vi "bats.parser.hostToFpga.testRunner.vi"(9 "Test.Messages":variant[](array[variant]), 10 "Expected OrderBook.Command[]":T1[](array[typedef])) -> (0 "Failures.Count":i32=1, 1 "Actual [str]":string[](array[string]), 2 "Passed":bool, 3 "OrderBook.Command[]":T1[](array[typedef]), 4 "Debug":u64[](array[numeric]) format="%.0x", 5 "Expected [str]":string[](array[string]))   [LabVIEW 2020]
uses:
  Market.Data.Common/fpga/orderbook.command.ctl
  Market.Data.Common/fpga/orderbook.command.type.ctl
  <vilib>/rvi/interface/RandomDataEmulation/nirviRandomDataOpen.vi
  <vilib>/rvi/interface/common/niFpgaCacheSessionInfoDynamic.vi
  <vilib>/Utility/error.llb/Error Cluster From Error Code.vi
  <vilib>/rvi/errors/niLvFpgaAdjustHostInterfaceError.vi
  <vilib>/FPGAPlugInAG/Dynamic/niLvFpga_Close_Dynamic.vi
  <vilib>/rvi/interface/nirviOpenFPGA/nirviOpenFPGA.xnode
  fpga/bats.parser.test.vi
  <vilib>/rvi/interface/nirviReadWriteControl/nirviReadWriteControl.xnode
  <vilib>/rvi/interface/nirviMethod/nirviMethod.xnode
  <vilib>/rvi/interface/nirviCloseFPGA/nirviCloseFPGA.xnode
  <vilib>/rvi/errors/niLvFpgaMergeErrorWithErrorCode.vi
  <vilib>/FPGAPlugInAG/Dynamic/niLvFpga_ReadFifo_Dynamic.vi
  <vilib>/rvi/interface/Simulation/niFpgaSimulationCallBeginRW.vi
  Market.Data.Common/host/fpganow.common.host.lvlib
  NiFpgaLv.dll
  <vilib>/FPGAPlugInAG/Dynamic/niLvFpga_WriteFifo_Dynamic.vi
  Market.Data.Common/fpga/fpganow.common.fpga.lvlib
panel:
  out "size(s)":i32
  out "Words.Out":u16[](array[numeric]) format="%.0x"
  out "Data.size":i32=16
  in  "Execute?":bool=TRUE
  out "Data":u64[](array[numeric]) format="%.0x"
  out "error out":errorcluster
  in  "error in":errorcluster
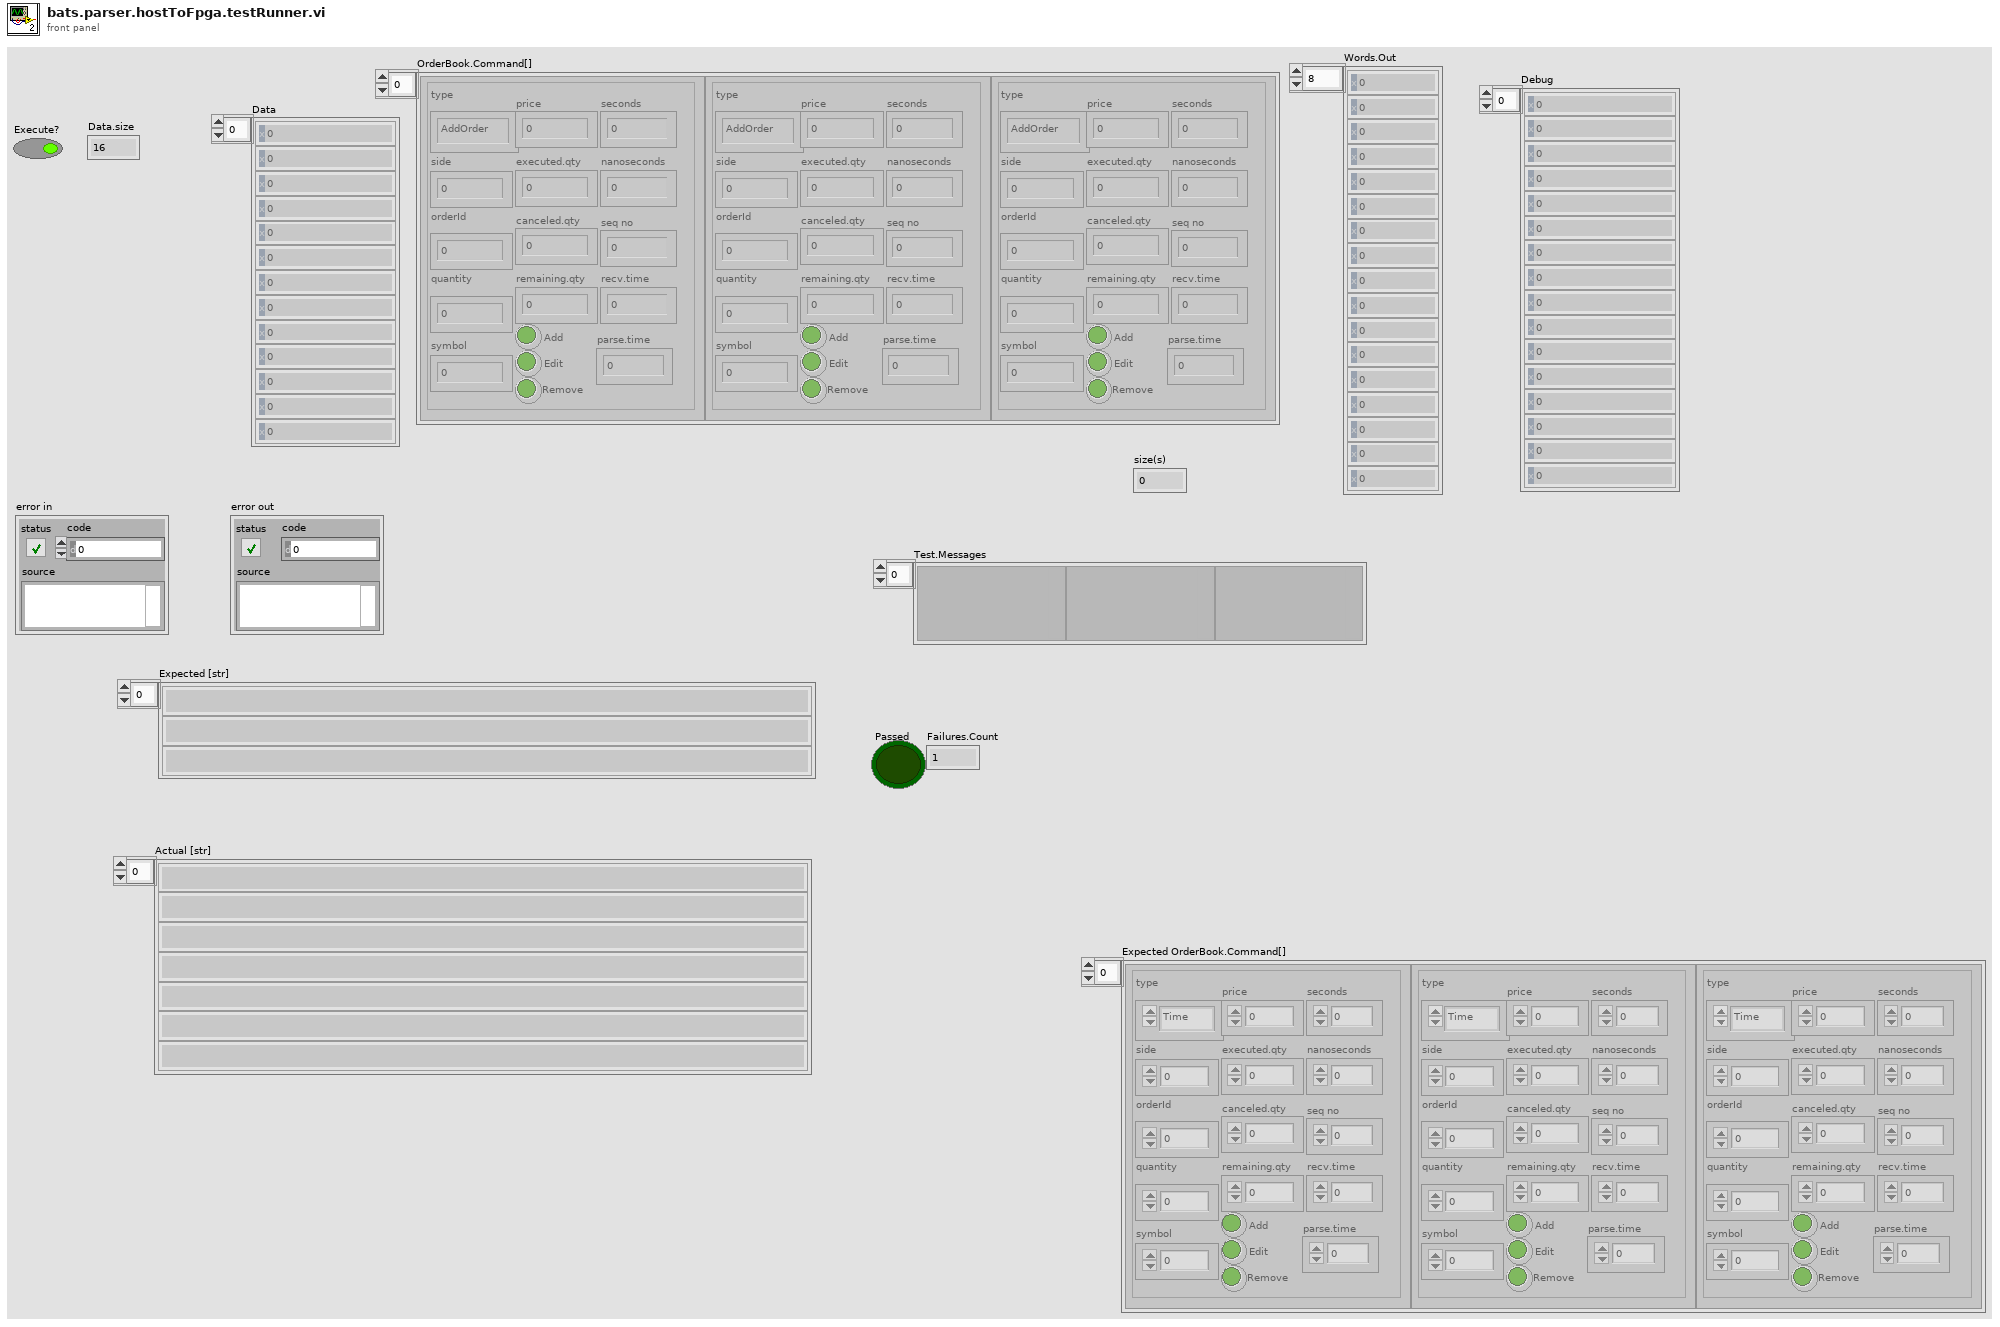
[diagram p1: front panel]
types:
  T1 = typedef "fpganow.common.fpga.lvlib/orderbook.command.ctl" = cluster{"type":T2, "side":u8, "orderId ":u64, "quantity":u32, "symbol":u64, "price":u64, "executed.qty":u32, "canceled.qty":u32, "remaining.qty":u32, "seconds":u64, "nanoseconds":u64, "Add":bool, "Edit":bool, "Remove":bool, "seq no":u32, "recv.time":u64, "parse.time":u64}
  T2 = typedef "fpganow.common.fpga.lvlib/orderbook.command.type.ctl" = enum8{"Time", "AddOrder", "OrderExecuted", "OrderExecutedAtPrice", "ReduceSize", "ModifyOrder", "DeleteOrder", "Get.Everything", "Get.All.Orders", "Get.Top"}
  T3 = cluster{"type":bool, "side":bool, "orderId ":bool, "quantity":bool, "symbol":bool, "price":bool, "executed.qty":bool, "canceled.qty":bool, "remaining.qty":bool, "seconds":bool, "nanoseconds":bool, "Add":bool, "Edit":bool, "Remove":bool, "seq no":bool, "recv.time":bool, "parse.time":bool}
  T4 = cluster{"Index":i32, "x = y?":cluster{"type":bool, "side":bool, "orderId ":bool, "quantity":bool, "symbol":bool, "price":bool, "executed.qty":bool, "canceled.qty":bool, "remaining.qty":bool, "seconds":bool, "nanoseconds":bool, "Add":bool, "Edit":bool, "Remove":bool, "seq no":bool, "recv.time":bool, "parse.time":bool}}
  T5 = cluster{"Index":i32, "x = y?":cluster{"type":bool, "side":bool, "orderId ":bool, "quantity":bool, "symbol":bool, "price":bool, "executed.qty":bool, "canceled.qty":bool, "remaining.qty":bool, "seconds":bool, "nanoseconds":bool, "Add":bool, "Edit":bool, "Remove":bool, "seq no":bool, "recv.time":bool, "parse.time":bool}}[]
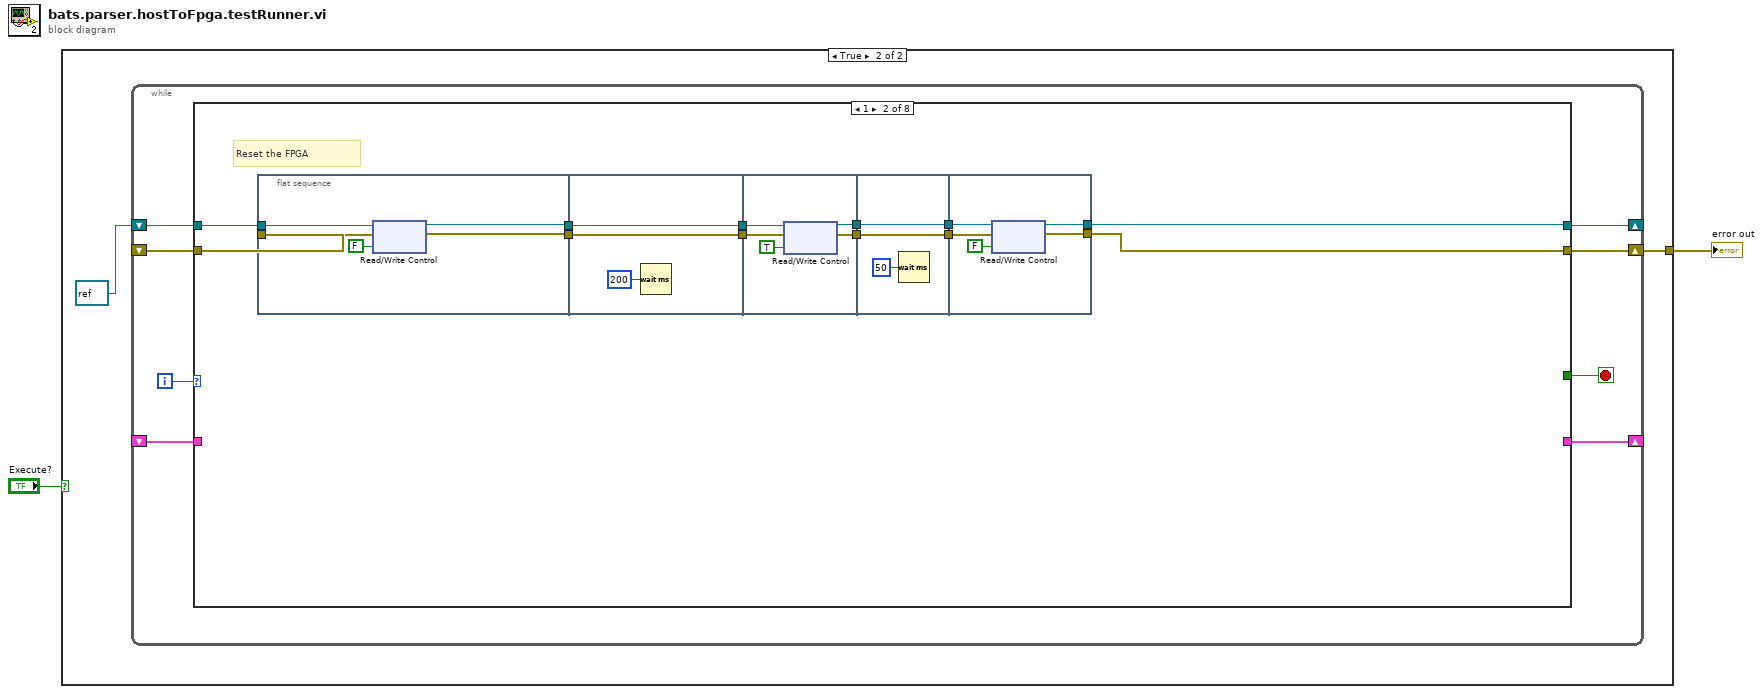
[diagram p0: block diagram]
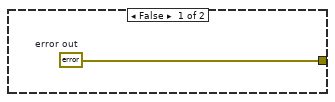
[diagram p2: hidden frame]
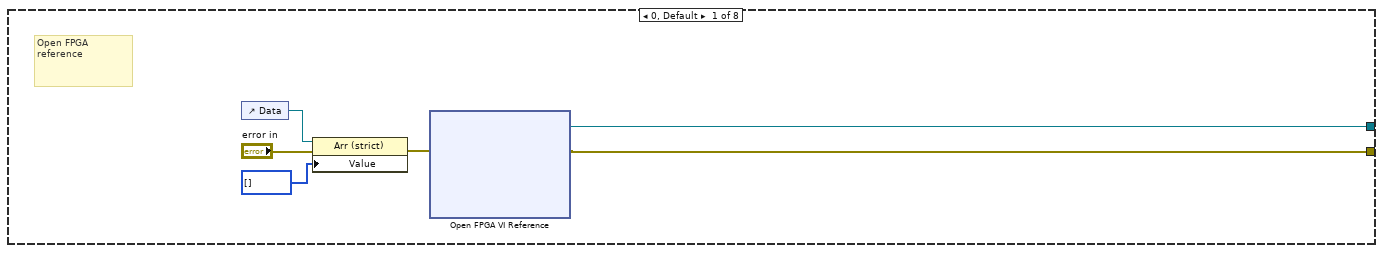
[diagram p3: hidden frame]
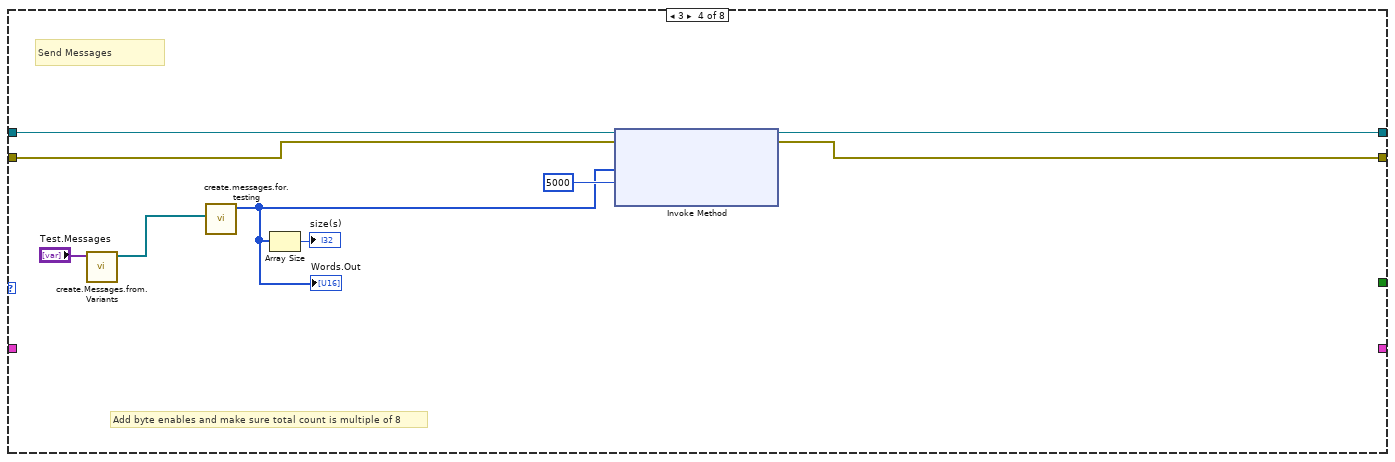
[diagram p5: hidden frame]
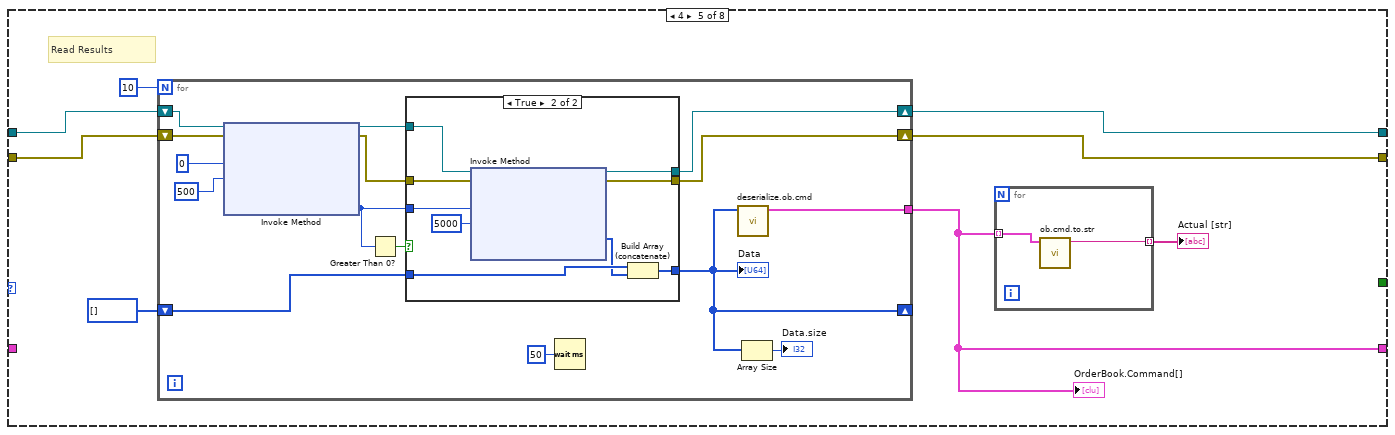
[diagram p6: hidden frame]
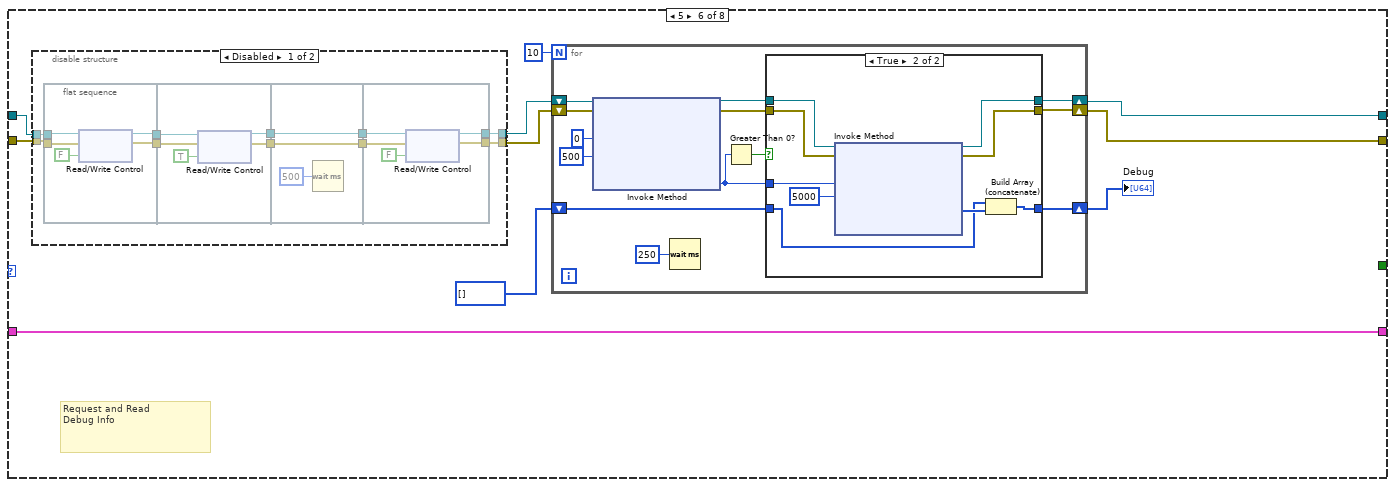
[diagram p8: hidden frame]
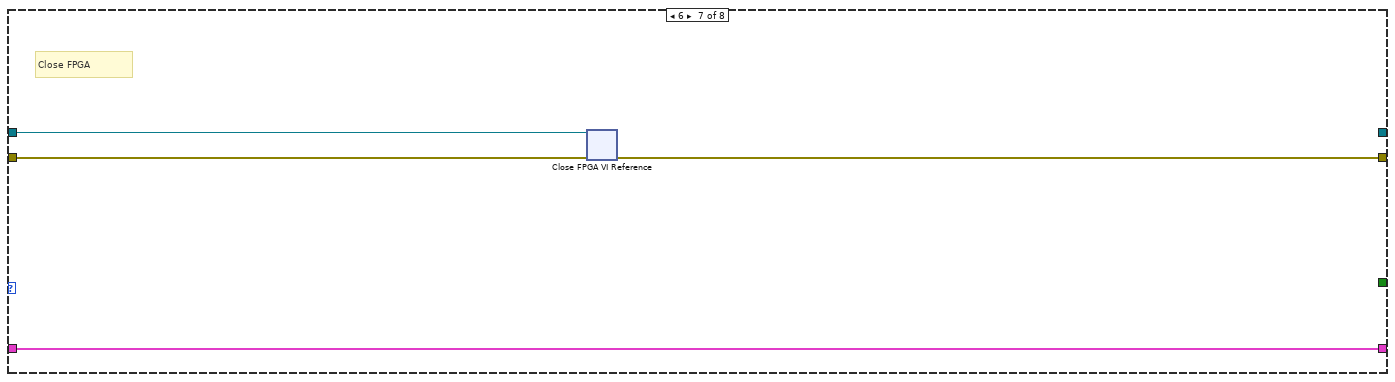
[diagram p11: hidden frame]
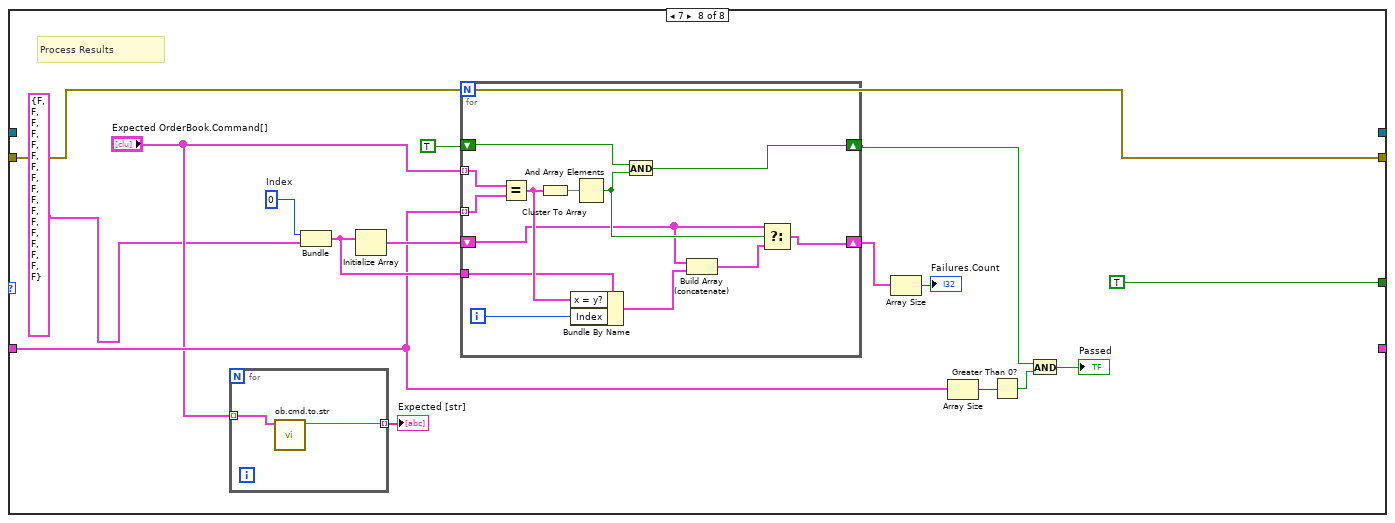
[diagram p12: hidden frame]
diagram:
  n1 = case shown="True" "Execute?" {
    tunnel: [w3 w5] -> w2
    frame False {
      w3 = errorcluster {"status"=FALSE, "code"=0, "source"=""}  # error out
    }
    frame True {
      n2 = while {
        shift-right: [w11] -> _
        shift-left: refnum<k20> refnum ("FPGA VI Reference Out") -> [w9]
        shift-right: [w10] -> w5
        shift-left: _ -> [w8]
        shift-right: [w7] -> _
        shift-left: _ -> [w6]
        i -> [w13]
        stop <- w12 stop-if-true
        n3 = case shown="1" w13 {
          tunnel: [_ _ _ _ _ _ _ TRUE] -> w12
          tunnel: [w14 w24 w54 w60 w66 w105 _ _] -> w11
          tunnel: [w15 w25 w53 w59 w67 w106 w169 w173] -> w10
          tunnel: w9 -> [_ w27 w54 w62 w69 w109 w168 _]
          tunnel: w8 -> [_ w26 w53 w61 w68 w110 w167 w173]
          tunnel: [_ _ _ _ w65 w101 w166 _] -> w7
          tunnel: w6 -> [_ _ _ _ _ w101 w166 w174]
          frame 0, Default {
            # "Open FPGA\nreference"
            n4 = control-ref of="Data"() -> (w17:refnum<vi>)
            n5 = property class="Arr (strict)"(reference=w17, error in="error in", "Value"=u8[] []) -> (error out=w19:errorcluster)  [unwired: 1 out]
            n6 = xnode ("Open FPGA VI Reference")("error in"=w19) -> ("FPGA VI Reference Out"=w14:refnum<k20>, "error out"=w15:errorcluster)  [unwired: 1 in]
          }
          frame 1 {
            # "Reset the FPGA"
            n7 = flat-sequence {
              tunnel: [w35] -> w23
              tunnel: [w36] -> w21
              tunnel: w27 -> [w33]
              tunnel: w26 -> [w34]
              tunnel: w23 -> [w39]
              tunnel: [w39] -> w22
              tunnel: w21 -> [w38]
              tunnel: [w38] -> w20
              tunnel: [w43] -> w31
              tunnel: [w42] -> w30
              tunnel: w22 -> [w41]
              tunnel: w20 -> [w40]
              tunnel: [w47] -> w29
              tunnel: w31 -> [w47]
              tunnel: w30 -> [w46]
              tunnel: [w46] -> w28
              tunnel: w29 -> [w51]
              tunnel: w28 -> [w50]
              tunnel: [w49] -> w25
              tunnel: [w48] -> w24
              frame #0 {
                n8 = xnode "Read/Write Control"("FPGA VI Reference In"=w33, "error in"=w34, "reset"=FALSE) -> ("FPGA VI Reference Out"=w36:refnum<k20>, "error out"=w35:errorcluster)
              }
              frame #1 {
                n9 = Wait (ms)(milliseconds to wait=u32 200) -> ()  [unwired: 1 out]
              }
              frame #2 {
                n10 = xnode "Read/Write Control"("FPGA VI Reference In"=w40, "error in"=w41, "reset"=TRUE) -> ("FPGA VI Reference Out"=w42:refnum<k20>, "error out"=w43:errorcluster)
              }
              frame #3 {
                n11 = Wait (ms)(milliseconds to wait=u32 50) -> ()  [unwired: 1 out]
              }
              frame #4 {
                n12 = xnode "Read/Write Control"("FPGA VI Reference In"=w50, "error in"=w51, "reset"=FALSE) -> ("FPGA VI Reference Out"=w48:refnum<k20>, "error out"=w49:errorcluster)
              }
            }
          }
          frame 2 {
            # "Memory Configuration"
          }
          frame 3 {
            # "Add byte enables and make sure total count is multiple of 8"
            # "Send Messages"
            n13 = call "create.Messages.from.Variants.vi"("Messages.Variant"="Test.Messages") -> ("Messages"=w56:refnum<class "MessageBase.lvclass">[])  [unwired: 10 in]
            n14 = call "create.messages.for.testing.vi"("Message.to.Create"=w56) -> ("Words.Out"=w58:u16[])  [unwired: 10 in]
            "Words.Out" <- w58
            n15 = Array Size(array=w58) -> (size(s)=→"size(s)":i32)
            n16 = xnode "Invoke Method"("FPGA VI Reference In"=w62, "error in"=w61, "Data"=w58, "Timeout (ms)"=5000) -> ("FPGA VI Reference Out"=w60:refnum<k20>, "error out"=w59:errorcluster)  [unwired: 1 out]
          }
          frame 4 {
            # "Read Results"
            n17 = for {
              N: 10 -> [_]
              shift-right: [w76] -> _
              shift-left: u64[] [] -> [w81]
              shift-right: [w80] -> w66
              shift-left: w69 -> [w88]
              shift-right: [w79] -> w67
              shift-left: w68 -> [w87]
              tunnel: [w74] -> w65
              n18 = xnode "Invoke Method"("FPGA VI Reference In"=w88, "error in"=w87, "Number of Elements"=u32 0, "Timeout (ms)"=500) -> ("FPGA VI Reference Out"=w82:refnum<k20>, "error out"=w78:errorcluster, "Elements Remaining"=w83:u32)  [unwired: 1 out]
              n19 = Greater Than 0?(x=w83) -> (x > 0?=w84:bool)
              n20 = case shown="True" w84 {
                tunnel: w83 -> [_ w100]
                tunnel: w82 -> [w90 w98]
                tunnel: [w91 w95] -> w76
                tunnel: w81 -> [w91 w97]
                tunnel: [w90 w94] -> w80
                tunnel: [w89 w93] -> w79
                tunnel: w78 -> [w89 w92]
                frame False {
                }
                frame True {
                  n21 = xnode "Invoke Method"("FPGA VI Reference In"=w98, "error in"=w92, "Number of Elements"=w100, "Timeout (ms)"=5000) -> ("FPGA VI Reference Out"=w94:refnum<k20>, "error out"=w93:errorcluster, "Data"=w96:u64[])  [unwired: 1 out]
                  n22 = Build Array (concatenate)(w97, w96) -> (w95:u64[])
                }
              }
              "Data" <- w76
              n23 = Wait (ms)(milliseconds to wait=u32 50) -> ()  [unwired: 1 out]
              n24 = call "deserialize.ob.cmd.vi"("DataIn"=w76) -> ("OrderBook.Command[]"=w74:T1[])  [unwired: 10 in]
              n25 = Array Size(array=w76) -> (size(s)=→"Data.size":i32)
            }
            "OrderBook.Command[]" <- w65
            n26 = for {
              tunnel: w65 -> [w73] mode=indexing
              tunnel: [w72] -> w64 mode=indexing
              n27 = call "ob.cmd.to.str.vi"("orderbook.command"=w73) -> ("string"=w72:string)  [unwired: 10 in]
            }
            "Actual [str]" <- w64
          }
          frame 5 {
            # "Request and Read\nDebug Info"
            n28 = disable-structure shown="Disabled" {
              disable-tunnel: w110 -> [w114 w139]
              disable-tunnel: w109 -> [w113 w140]
              disable-tunnel: [w112 w140] -> w108
              disable-tunnel: [w111 w139] -> w107
              frame Disabled {
                n29 = flat-sequence {
                  tunnel: w113 -> [w122]
                  tunnel: w114 -> [w123]
                  tunnel: [w124] -> w120
                  tunnel: [w125] -> w119
                  tunnel: [w129] -> w118
                  tunnel: [w128] -> w117
                  tunnel: w120 -> [w127]
                  tunnel: w119 -> [w126]
                  tunnel: [w133] -> w116
                  tunnel: w118 -> [w133]
                  tunnel: w117 -> [w132]
                  tunnel: [w132] -> w115
                  tunnel: w116 -> [w137]
                  tunnel: w115 -> [w136]
                  tunnel: [w135] -> w111
                  tunnel: [w134] -> w112
                  frame #0 {
                    n30 = xnode "Read/Write Control"("FPGA VI Reference In"=w122, "error in"=w123, "debug"=FALSE ("reset")) -> ("FPGA VI Reference Out"=w125:refnum<k20>, "error out"=w124:errorcluster)
                  }
                  frame #1 {
                    n31 = xnode "Read/Write Control"("FPGA VI Reference In"=w126, "error in"=w127, "debug"=TRUE ("reset")) -> ("FPGA VI Reference Out"=w128:refnum<k20>, "error out"=w129:errorcluster)
                  }
                  frame #2 {
                    n32 = Wait (ms)(milliseconds to wait=u32 500) -> ()  [unwired: 1 out]
                  }
                  frame #3 {
                    n33 = xnode "Read/Write Control"("FPGA VI Reference In"=w136, "error in"=w137, "debug"=FALSE ("reset")) -> ("FPGA VI Reference Out"=w134:refnum<k20>, "error out"=w135:errorcluster)
                  }
                }
              }
              frame Enabled {
              }
            }
            n34 = for {
              N: 10 -> [_]
              shift-right: [w147] -> w105
              shift-left: w108 -> [w153]
              shift-right: [w146] -> w106
              shift-left: w107 -> [w152]
              shift-right: [w148] -> w104
              shift-left: u64[] [] -> [w142]
              n35 = xnode "Invoke Method"("FPGA VI Reference In"=w153, "error in"=w152, "Number of Elements"=u32 0, "Timeout (ms)"=500) -> ("FPGA VI Reference Out"=w145:refnum<k20>, "error out"=w144:errorcluster, "Elements Remaining"=w143:u32)  [unwired: 1 out]
              n36 = Wait (ms)(milliseconds to wait=u32 250) -> ()  [unwired: 1 out]
              n37 = Greater Than 0?(x=w143) -> (x > 0?=w149:bool)
              n38 = case shown="True" w149 {
                tunnel: [w154 w164] -> w148
                tunnel: [w156 w163] -> w147
                tunnel: [w155 w162] -> w146
                tunnel: w145 -> [w156 w161]
                tunnel: w144 -> [w155 w160]
                tunnel: w143 -> [_ w159]
                tunnel: w142 -> [w154 w157]
                frame False {
                }
                frame True {
                  n39 = xnode "Invoke Method"("FPGA VI Reference In"=w161, "error in"=w160, "Number of Elements"=w159, "Timeout (ms)"=5000) -> ("FPGA VI Reference Out"=w163:refnum<k20>, "error out"=w162:errorcluster, "Data"=w165:u64[])  [unwired: 1 out]
                  n40 = Build Array (concatenate)(w157, w165) -> (w164:u64[])
                }
              }
            }
            "Debug" <- w104
          }
          frame 6 {
            # "Close FPGA"
            n41 = xnode "Close FPGA VI Reference"("FPGA VI Reference In"=w168, "error in"=w167) -> ("error out"=w169:errorcluster)
          }
          frame 7 {
            w176 = 0  # Index
            # "Process Results"
            n42 = for {
              tunnel: "Expected OrderBook.Command[]" -> [w187] mode=indexing
              tunnel: [w186] -> w171 mode=indexing
              n43 = call "ob.cmd.to.str.vi"("orderbook.command"=w187) -> ("string"=w186:string)  [unwired: 10 in]
            }
            "Expected [str]" <- w171
            n44 = Bundle("Index"=w176, "x = y?"=T3 {"type"=FALSE, "side"=FALSE, "orderId "=FALSE, "quantity"=FALSE, "symbol"=FALSE, "price"=FALSE, "executed.qty"=FALSE, "canceled.qty"=FALSE, "remaining.qty"=FALSE, "seconds"=FALSE, "nanoseconds"=FALSE, "Add"=FALSE, "Edit"=FALSE, "Remove"=FALSE, "seq no"=FALSE, "recv.time"=FALSE, "parse.time"=FALSE}) -> (w178:T4)  [unwired: 1 in]
            n45 = Initialize Array(w178) -> (w177:T5)  [unwired: 1 in]
            n46 = for {
              tunnel: "Expected OrderBook.Command[]" -> [w200] mode=indexing
              tunnel: w174 -> [w199] mode=indexing
              shift-right: [w197] -> w184
              shift-left: TRUE -> [w198]
              shift-right: [w194] -> w179
              shift-left: w177 -> [w189]
              tunnel: w178 -> [w192]
              i -> [w191]
              n47 = Equal?(x=w200, y=w199) -> (x = y?=w193:T3)
              n48 = Cluster To Array(cluster=w193) -> (array=w196:bool[])
              n49 = Bundle By Name(cluster=w192, "x = y?"=w193, "Index"=w191) -> (w190:T4)
              n50 = And Array Elements(Boolean array=w196) -> (logical AND=w195:bool)
              n51 = And(x=w198, y=w195) -> (x .and. y?=w197:bool)
              n52 = Build Array (concatenate)(w189, w190) -> (w188:T5)
              n53 = Select(t=w189, s=w195, f=w188) -> (s? t:f=w194:T5)
            }
            n54 = Array Size(array=w179) -> (size(s)=→"Failures.Count":i32)
            n55 = Array Size(array=w174) -> (size(s)=w181:i32)
            n56 = Greater Than 0?(x=w181) -> (x > 0?=w182:bool)
            n57 = And(x=w184, y=w182) -> (x .and. y?=→"Passed":bool)
          }
        }
      }
    }
  }
  "error out" <- w2
